vi "FullAlign.vi"(0 "Joystick 0":dbl, 5 "Joystick 1":dbl, 7 "Distance":dbl=23.73829999999998, 9 "Angle":dbl=57.28800997198897) -> (4 "Right Motor":dbl, 6 "Left Motor":dbl=-0.0, 15 "In Range?":bool)   [LabVIEW 2016]
panel:
  out "Sees Target?":bool=TRUE
  in  "Button":bool=TRUE
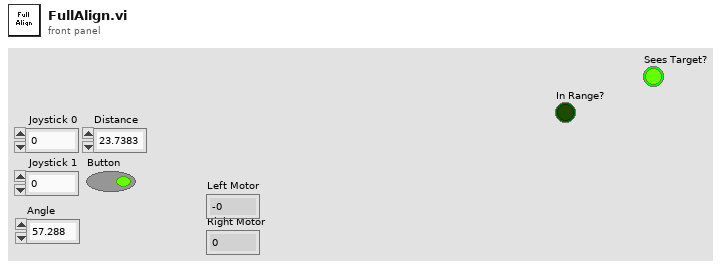
[diagram p1: front panel]
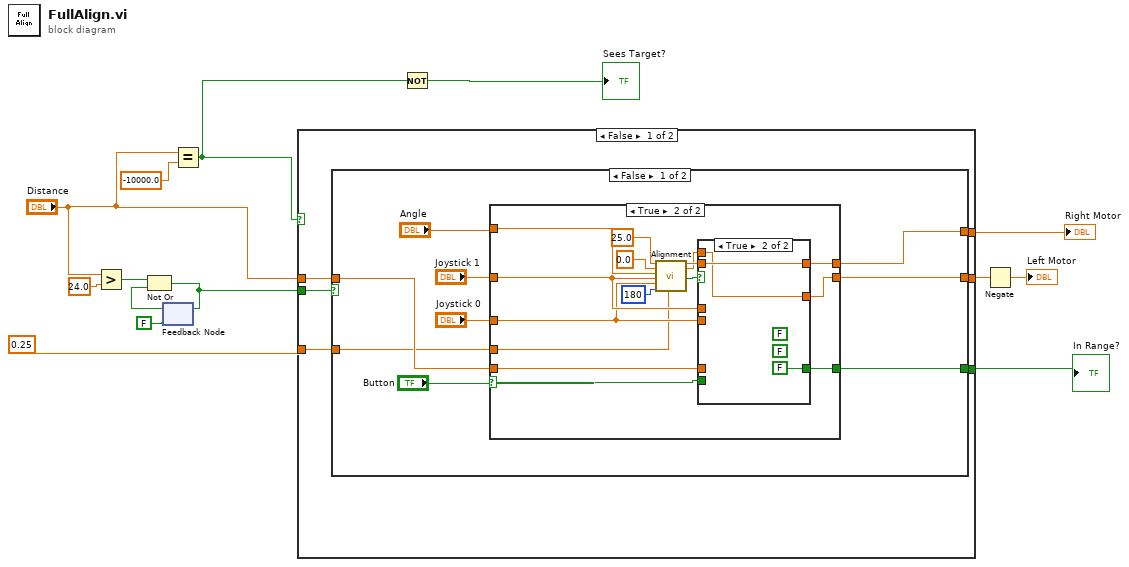
[diagram p0: block diagram]
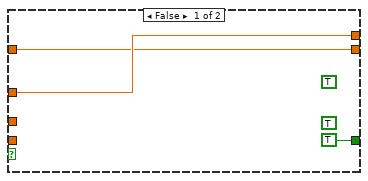
[diagram p2: hidden frame]
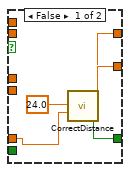
[diagram p3: hidden frame]
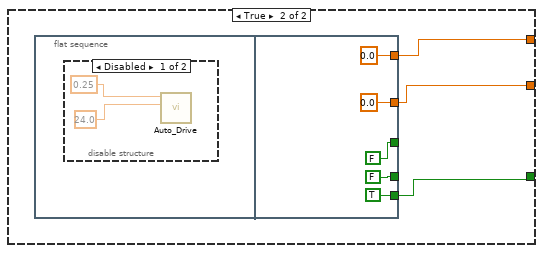
[diagram p4: hidden frame]
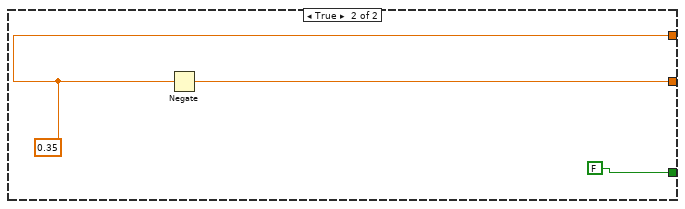
[diagram p6: hidden frame]
diagram:
  n1 = Greater?(x="Distance", y=24.0) -> (0:w11:bool)
  n2 = feedback #1(FALSE) -> (w12:bool)
  n3 = Not Or(1:w12, 2:w11) -> (0:w10:bool)
  n4 = feedback-in #1(w10) -> ()
  n5 = Equal?(x="Distance", y=-10000.0) -> (x = y?=w4:bool)
  n6 = case shown="False" w4 {
    tunnel: w10 -> [w20 _]
    tunnel: [w19 w66] -> w6
    tunnel: [w18 w67] -> w9
    tunnel: [w17 FALSE] -> w8
    tunnel: "Distance" -> [w16 _]
    tunnel: 0.25 -> [w15 _]
    frame False {
      n7 = case shown="False" w20 {
        tunnel: w16 -> [w25 _]
        tunnel: [w24 w57] -> w19
        tunnel: [w23 w56] -> w18
        tunnel: [w22 w58] -> w17
        tunnel: w15 -> [w21 _]
        frame False {
          n8 = case shown="True" "Button" {
            selector: "Button" -> [_ w39]
            tunnel: "Joystick 1" -> [w31 w42]
            tunnel: "Joystick 0" -> [w32 w41]
            tunnel: [w31 w47] -> w23
            tunnel: [w32 w46] -> w24
            tunnel: "Angle" -> [_ w44]
            tunnel: [TRUE w38] -> w22
            tunnel: w25 -> [_ w37]
            tunnel: w21 -> [_ w35]
            frame False {
              (unwired) TRUE
              (unwired) TRUE
            }
            frame True {
              n9 = call "Alignment.vi"("Range"=25.0, "Camera Feedback"=0.0, "Target"=w44, "POV"=w42, "Max Error"=w41, "Effort Addition"=180, "Turn_Gain"=w35) -> ("Right Motor"=w34:dbl, "Left Motor"=w33:dbl, "LeftAndRight?"=w40:bool)  [unwired: 10 in]
              n10 = case shown="True" w40 {
                tunnel: w42 -> [_ _]
                tunnel: w41 -> [_ _]
                tunnel: [w51 w53] -> w47
                tunnel: [w50 w55] -> w46
                tunnel: w39 -> [_ _]
                tunnel: w34 -> [_ w55]
                tunnel: [w48 FALSE] -> w38
                tunnel: w37 -> [w49 _]
                tunnel: w33 -> [_ w53]
                frame False {
                  n11 = call "CorrectDistance.vi"("CenterPoint"=24.0, "Distance"=w49) -> ("In Range?"=w48:bool, "Right Motor"=w50:dbl, "Left Motor"=w51:dbl)  [unwired: 23 in]
                }
                frame True {
                  (unwired) FALSE
                  (unwired) FALSE
                }
              }
            }
          }
        }
        frame True {
          n12 = flat-sequence {
            tunnel: [FALSE] -> _
            tunnel: [FALSE] -> _
            tunnel: [TRUE] -> w58
            tunnel: [0.0] -> w57
            tunnel: [0.0] -> w56
            frame #0 {
              n13 = disable-structure shown="Disabled" {
                frame Disabled {
                  n14 = call "Auto_Drive.vi"("distance"=24.0, "Drive Effort"=0.25) -> ()  [unwired: 10 in]
                }
                frame Enabled {
                }
              }
            }
            frame #1 {
            }
          }
        }
      }
    }
    frame True {
      w66 = 0.35
      n15 = Negate(x=w66) -> (-x=w67:dbl)
    }
  }
  "Right Motor" <- w6
  "In Range?" <- w8
  n16 = Not(x=w4) -> (.not. x?=→"Sees Target?":bool)
  n17 = Negate(x=w9) -> (-x=→"Left Motor":dbl)
